vi "new Remote Terminal.vi"(8 "error in":errorcluster, 10 "Remote Terminal Config":T1={"rtAddress"=0, "rtMode"=0, "initialSwd"=[0, 0], "noBuild"=FALSE, "autoBusy"=FALSE, "dynamicBC"=FALSE, "clearSwdImmediate"=FALSE, "busEnable"=2, "dataWipe"=0, "syncMode"=0, "responseMode"=1, "responseTime"=9.0} {"responseMode" items=["Selective", "All"]; "syncMode" items=["Zeroes", "Item123", "CWD", "None"]; "dataWipe" items=["A", "B", "AB", "None"]; "busEnable" items=["A", "B", "AB", "None"]; "rtMode" items=["Simulate", "Monitor", "Disable"]}, 11 "name":string) -> (0 "error out":errorcluster, 3 "remoteTerminal out":refnum<k24>)   [LabVIEW 2020, in "Ballard_1553_Hardware_ni.lvlib"]
uses:
  Ballard_1553_Hardware_ni.lvlib
  C:/Users/Administrator/Desktop/GIT/Ballard-MIL-STD-1553-Custom-Device/Source/System Explorer/SubVIs/Parse XML Ballard/1.2/BTIXML_SerDes.dll
  Ballard-MIL-STD-1553-Custom-Device/Source/System Explorer/SubVIs/Parse XML Ballard/1.2/BTIXML_SerDes.dll
  _typedefs/RemoteTerminal_type.ctl
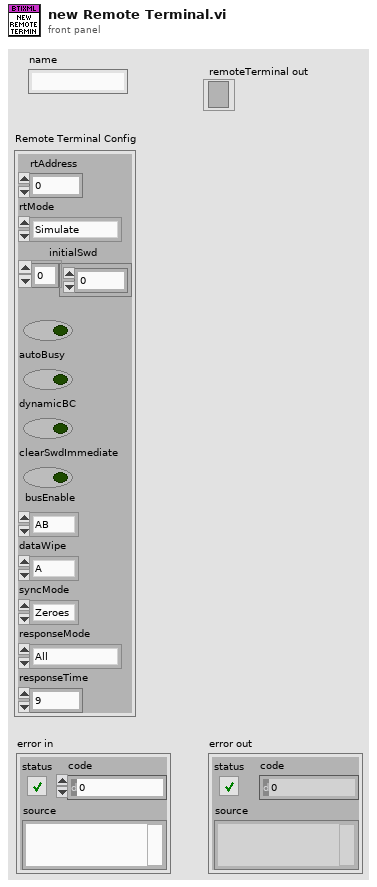
[diagram p1: front panel]
types:
  T1 = typedef "Ballard_1553_Hardware_ni.lvlib/RemoteTerminal_type.ctl" = cluster{"rtAddress":i8, "rtMode":i32, "initialSwd":u8[], "noBuild":bool, "autoBusy":bool, "dynamicBC":bool, "clearSwdImmediate":bool, "busEnable":i32, "dataWipe":i32, "syncMode":i32, "responseMode":i32, "responseTime":dbl}
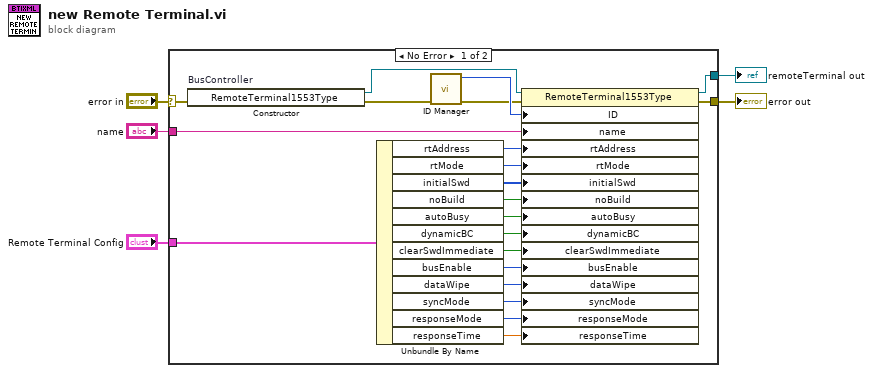
[diagram p0: block diagram]
diagram:
  n1 = case shown="No Error" "error in" {
    selector: "error in" -> [w26 w27]
    tunnel: [w25 w27] -> w4
    tunnel: [w24 _] -> w2
    tunnel: "Remote Terminal Config" -> [w19 _]
    tunnel: "name" -> [w6 _]
    frame No Error {
      n2 = constructor on="BusController" class="RemoteTerminal1553Type"(error in=w26) -> (reference out=w23:refnum<k24>, error out=w22:errorcluster)  [unwired: 2 in, 1 out]
      n3 = Unbundle By Name(w19) -> ("rtAddress"=w18:i8, "rtMode"=w17:i32, "initialSwd"=w16:u8[], "noBuild"=w15:bool, "autoBusy"=w14:bool, "dynamicBC"=w13:bool, "clearSwdImmediate"=w12:bool, "busEnable"=w11:i32, "dataWipe"=w10:i32, "syncMode"=w9:i32, "responseMode"=w8:i32, "responseTime"=w7:dbl)
      n4 = call "ID Manager.vi"("error in"=w22) -> ("error out"=w20:errorcluster, "ID out"=w21:i32)  [unwired: 9 in]
      n5 = property class="RemoteTerminal1553Type"(reference=w23, error in=w20, "ID"=w21, "name"=w6, "rtAddress"=w18, "rtMode"=w17, "initialSwd"=w16, "noBuild"=w15, "autoBusy"=w14, "dynamicBC"=w13, "clearSwdImmediate"=w12, "busEnable"=w11, "dataWipe"=w10, "syncMode"=w9, "responseMode"=w8, "responseTime"=w7) -> (reference out=w24:refnum<k24>, error out=w25:errorcluster)
    }
    frame Error {
    }
  }
  "error out" <- w4
  "remoteTerminal out" <- w2
